vi "mod_AM SSB CE Demodulation (block processing).vi"(0 "input complex waveform":T5={"t0"=0.0, "dt"=1.0, "Y"=[]} {"Y" format="%.3f"; "dt" format="%^.2e"; "t0" format="%.4f"}, 1 "costas loop parameters":T2={"Alpha"=0.001, "Beta"=2e-05} {"Beta" format="%#_6p"; "Alpha" format="%#_6p"}, 5 "modulation index":dbl=1.0 format="%.2f", 7 "pilot extraction filter":T4={"taps"=81, "approx freq. (Hz)"=0.0, "search (+/- % of Fsampl) "=0.25}, 11 "error in (no error)":errorcluster, 12 "suppress carrier ? (F)":bool, 13 "reset? (T)":bool=TRUE) -> (4 "recovered message signal":dbl[](array[numeric]), 6 "measurements":T3, 8 "filter information":T1 {"Pilot rejection filter"."df" format="%.2p"; "Pilot rejection filter"."f0" format="%.2p"; "Pilot rejection filter"."Mag H(w)" format="%.2p"; "Pilot extraction filter"."df" format="%.2p"; "Pilot extraction filter"."f0" format="%.2p"; "Pilot extraction filter"."Mag H(w)" format="%.2p"}, 15 "error out":errorcluster)   [LabVIEW 2020, in "niAMT.lvlib"]
uses:
  <vilib>/addons/Modulation/niAMT.lvlib
  <vilib>/addons/Modulation/Analog/controls/Complex Data Waveform.ctl
  <vilib>/addons/Modulation/Analog/controls/mod_AM pilot extraction filter.ctl
  <vilib>/addons/Modulation/Analog/controls/mod_AM Measurements.ctl
  <vilib>/addons/Modulation/Analog/controls/mod_Costas loop parameters.ctl
  <vilib>/addons/Modulation/Analog/controls/mod_AM pilot filter info.ctl
  <vilib>/Analysis/baseanly.llb/Mean (DBL).vi
  <vilib>/addons/Modulation/Analog/MT Upconvert Baseband (Real).vi
  <vilib>/Analysis/0measdsp.llb/Scaled Time Domain Window (DBL).vi
  <vilib>/Analysis/NI_AALPro.lvlib
  <vilib>/Analysis/NI_AALBase.lvlib
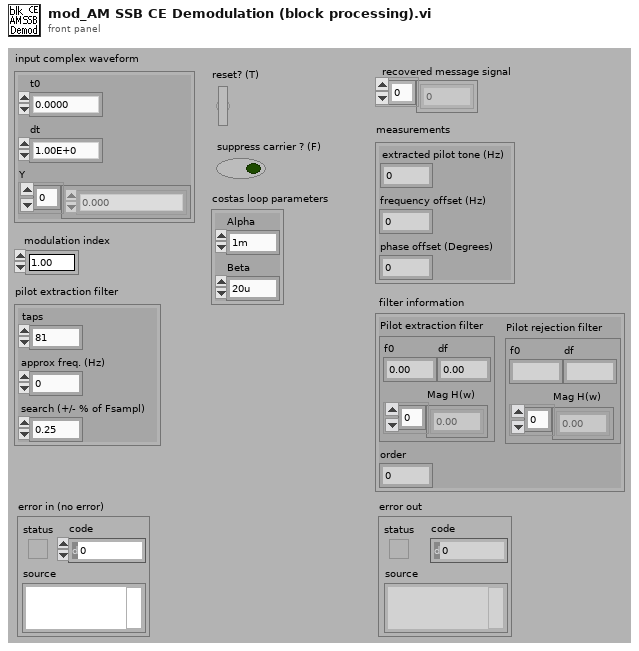
[diagram p1: front panel]
types:
  T1 = typedef "niAMT.lvlib/mod_AM pilot filter info.ctl" = cluster{"Pilot extraction filter":cluster{"f0":dbl, "df":dbl, "Mag H(w)":dbl[]}, "order":i32, "Pilot rejection filter":cluster{"f0":dbl, "df":dbl, "Mag H(w)":dbl[]}}
  T2 = typedef "niAMT.lvlib/mod_Costas loop parameters.ctl" = cluster{"Alpha":dbl, "Beta":dbl}
  T3 = typedef "niAMT.lvlib/mod_AM Measurements.ctl" = cluster{"extracted pilot tone (Hz)":dbl, "phase offset (Degrees)":dbl, "frequency offset (Hz)":dbl}
  T4 = typedef "niAMT.lvlib/mod_AM pilot extraction filter.ctl" = cluster{"taps":i32, "approx freq. (Hz)":dbl, "search (+/- % of Fsampl) ":dbl}
  T5 = typedef "niAMT.lvlib/Complex Data Waveform.ctl" = cluster{"t0":dbl, "dt":dbl, "Y":cdb[]}
  T6 = enum16{"None ", "Hanning", "Hamming", "Blackman-Harris", "Exact Blackman", "Blackman", "Flat Top", "4 Term B-Harris ", "7 Term B-Harris", "Low Sidelobe"}
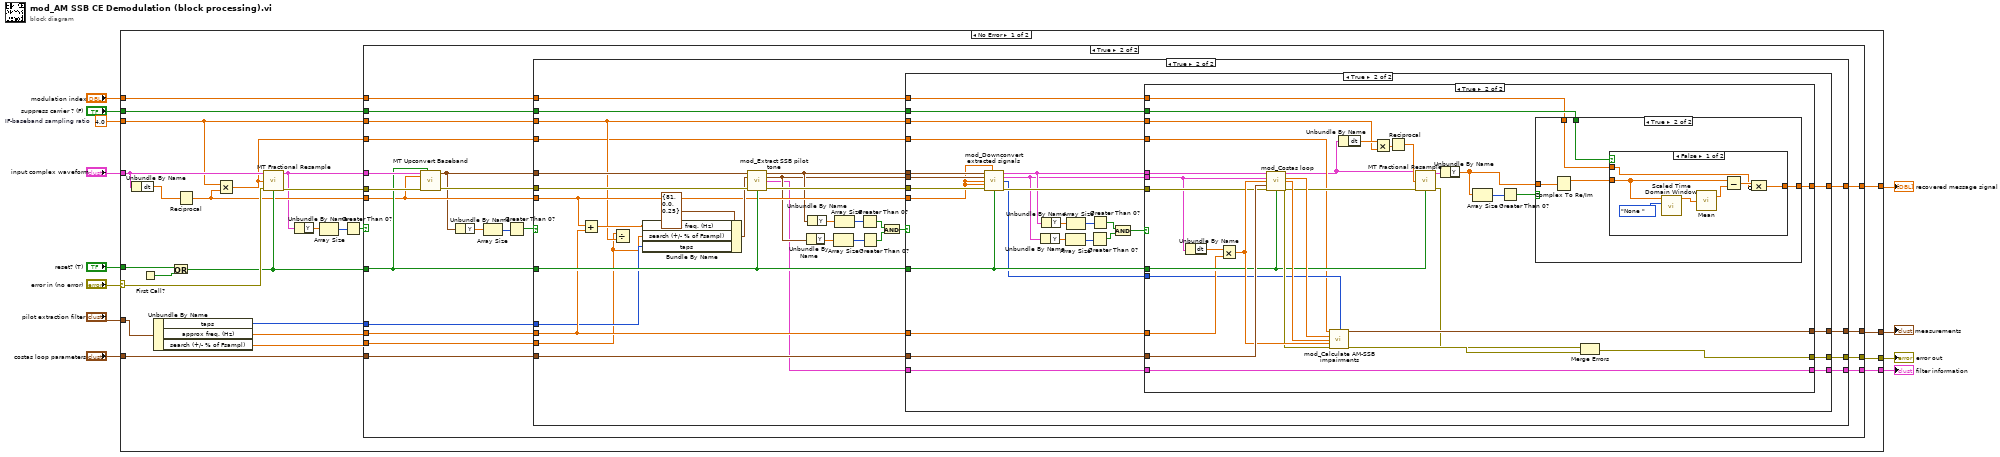
[diagram p0: block diagram]
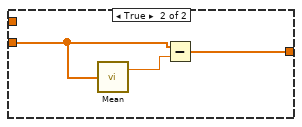
[diagram p7: hidden frame]
diagram:
  w2 = 4.0  # IF-baseband sampling ratio
  n1 = case shown="No Error" "error in (no error)" {
    selector: "error in (no error)" -> [w37 w165]
    tunnel: [w27 w165] -> w11
    tunnel: "input complex waveform" -> [w30 _]
    tunnel: "pilot extraction filter" -> [w32 _]
    tunnel: "reset? (T)" -> [w26 _]
    tunnel: "suppress carrier ? (F)" -> [w35 _]
    tunnel: "modulation index" -> [w34 _]
    tunnel: [w33 _] -> w4
    tunnel: "costas loop parameters" -> [w31 _]
    tunnel: [w29 _] -> w3
    tunnel: w2 -> [w19 _]
    tunnel: [w28 _] -> w1
    frame No Error {
      n2 = Unbundle By Name(w30) -> ("dt"=w21:dbl)
      n3 = First Call?() -> (First Call?: T/F=w24:bool)
      n4 = Unbundle By Name(w32) -> ("taps"=w17:i32, "approx freq. (Hz)"=w23:dbl, "search (+/- % of Fsampl)"=w22:dbl)
      n5 = Or(x=w26, y=w24) -> (x .or. y?=w25:bool)
      n6 = Reciprocal(x=w21) -> (1/x=w20:dbl)
      n7 = Multiply(x=w19, y=w20) -> (x*y=w18:dbl)
      n8 = call <vilib>:"MT Fractional Resample.vi"("input complex waveform"=w30, "desired sample rate (Hz)"=w18, "error in (no error)"=w37, "reset? (T)"=w25) -> ("output complex waveform"=w16:T5, "error out"=w36:errorcluster)  [unwired: 1 in, 9 out]
      n9 = Unbundle By Name(w16) -> ("Y"=w15:cdb[])
      n10 = Array Size(array=w15) -> (size(s)=w14:i32)
      n11 = Greater Than 0?(x=w14) -> (x > 0?=w13:bool)
      n12 = case shown="True" w13 {
        tunnel: w36 -> [w38 w59]
        tunnel: w35 -> [_ w58]
        tunnel: w34 -> [_ w57]
        tunnel: [_ w56] -> w33
        tunnel: w31 -> [_ w54]
        tunnel: w16 -> [_ w53]
        tunnel: [_ w52] -> w29
        tunnel: [_ w51] -> w28
        tunnel: [w38 w50] -> w27
        tunnel: w25 -> [_ w49]
        tunnel: w23 -> [_ w48]
        tunnel: w22 -> [_ w47]
        tunnel: w20 -> [_ w46]
        tunnel: w19 -> [_ w45]
        tunnel: w18 -> [_ w44]
        tunnel: w17 -> [_ w43]
        frame False {
          # "NOTE: Do not perform any processing, since input array sizes are zero-sized"
        }
        frame True {
          n13 = call-poly <vilib>:"MT Upconvert Baseband.vi"("baseband waveform (complex)"=w53, "reset? (F)"=w49, "carrier frequency (Hz)"=w46, "error in (no error)"=w59) -> ("passband waveform"=w41:waveform(dbl), "error out"=w55:errorcluster)  [unwired: 10 out]
          n14 = Unbundle By Name(w41) -> ("Y"=w40:dbl[])
          n15 = Array Size(array=w40) -> (size(s)=w42:i32)
          n16 = Greater Than 0?(x=w42) -> (x > 0?=w39:bool)
          n17 = case shown="True" w39 {
            tunnel: w58 -> [_ w90]
            tunnel: w57 -> [_ w89]
            tunnel: [_ w88] -> w56
            tunnel: w55 -> [w60 w87]
            tunnel: w54 -> [_ w86]
            tunnel: w41 -> [_ w84]
            tunnel: [_ w62] -> w52
            tunnel: [_ w83] -> w51
            tunnel: [w60 w82] -> w50
            tunnel: w49 -> [_ w79]
            tunnel: w48 -> [_ w78]
            tunnel: w47 -> [_ w61]
            tunnel: w46 -> [_ w77]
            tunnel: w45 -> [_ w76]
            tunnel: w44 -> [_ w75]
            tunnel: w43 -> [_ w73]
            frame False {
              # "NOTE: Do not perform any processing, since input array sizes are zero-sized"
            }
            frame True {
              n18 = Add(x=w77, y=w78) -> (x+y=w80:dbl)
              n19 = Divide(x=w61, y=w76) -> ()  [unwired: 1 out]
              n20 = Bundle By Name(cluster=T4 {"taps"=81, "approx freq. (Hz)"=0.0, "search (+/- % of Fsampl) "=0.25} ("pilot extraction filter"), "approx freq. (Hz)"=w80, "search (+/- % of Fsampl)"=w61, "taps"=w73) -> (w85:T4)
              n21 = call <vilib>:"mod_Extract SSB pilot tone.vi"("passband waveform"=w84, "pilot extraction filter"=w85, "error in (no error)"=w87, "reset? (T)"=w79) -> ("extracted AM modulated wfm (IF)"=w71:waveform(dbl), "extracted pilot tone wfm (IF)"=w69:waveform(dbl), "filter information"=w63:T1, "error out"=w81:errorcluster)  [unwired: 8 out]
              n22 = Unbundle By Name(w69) -> ("Y"=w70:dbl[])
              n23 = Unbundle By Name(w71) -> ("Y"=w72:dbl[])
              n24 = Array Size(array=w70) -> (size(s)=w67:i32)
              n25 = Array Size(array=w72) -> (size(s)=w68:i32)
              n26 = Greater Than 0?(x=w68) -> (x > 0?=w66:bool)
              n27 = Greater Than 0?(x=w67) -> (x > 0?=w65:bool)
              n28 = And(x=w66, y=w65) -> (x .and. y?=w64:bool)
              n29 = case shown="True" w64 {
                tunnel: w90 -> [_ w118]
                tunnel: w89 -> [_ w117]
                tunnel: [_ w116] -> w88
                tunnel: w86 -> [_ w115]
                tunnel: [_ w114] -> w83
                tunnel: [w91 w113] -> w82
                tunnel: w81 -> [w91 w112]
                tunnel: w71 -> [_ w111]
                tunnel: w69 -> [_ w110]
                tunnel: w79 -> [_ w109]
                tunnel: w78 -> [_ w107]
                tunnel: w77 -> [_ w105]
                tunnel: w76 -> [_ w104]
                tunnel: w75 -> [_ w103]
                tunnel: w63 -> [_ w101]
                tunnel: [_ w102] -> w62
                frame False {
                  # "NOTE: Do not perform any processing, since input array sizes are zero-sized"
                }
                frame True {
                  n30 = call <vilib>:"mod_Downconvert extracted signals.vi"("extracted AM modulated wfm (IF)"=w111, "carrier frequency"=w105, "extracted pilot tone wfm (IF)"=w110, "passband bandwidth (AM modulated wfm)"=w105, "passband bandwidth (pilot tone wfm)"=w105, "error in (no error)"=w112, "reset? (T)"=w109) -> ("extracted AM modulated signal (baseband)"=w98:cluster{"t0":dbl, "dt":dbl, "Y":cdb[]}, "extracted pilot tone (baseband)"=w95:cluster{"t0":dbl, "dt":dbl, "Y":cdb[]}, "downconversion filter length"=w106:i32, "error out"=w108:errorcluster)  [unwired: 5 out]
                  n31 = Unbundle By Name(w95) -> ("Y"=w96:cdb[])
                  n32 = Unbundle By Name(w98) -> ("Y"=w100:cdb[])
                  n33 = Array Size(array=w96) -> (size(s)=w97:i32)
                  n34 = Array Size(array=w100) -> (size(s)=w99:i32)
                  n35 = Greater Than 0?(x=w97) -> (x > 0?=w93:bool)
                  n36 = Greater Than 0?(x=w99) -> (x > 0?=w94:bool)
                  n37 = And(x=w94, y=w93) -> (x .and. y?=w92:bool)
                  n38 = case shown="True" w92 {
                    tunnel: w118 -> [_ w147]
                    tunnel: w117 -> [_ w146]
                    tunnel: [_ w145] -> w116
                    tunnel: w115 -> [_ w144]
                    tunnel: [_ w137] -> w114
                    tunnel: [w119 w134] -> w113
                    tunnel: w109 -> [_ w132]
                    tunnel: w108 -> [w119 w131]
                    tunnel: w107 -> [_ w130]
                    tunnel: w106 -> [_ w129]
                    tunnel: w104 -> [_ w128]
                    tunnel: w103 -> [_ w127]
                    tunnel: w98 -> [_ w126]
                    tunnel: w95 -> [_ w125]
                    tunnel: [_ w123] -> w102
                    tunnel: w101 -> [_ w123]
                    frame False {
                      # "NOTE: Do not perform any processing, since input array sizes are zero-sized"
                    }
                    frame True {
                      n39 = Unbundle By Name(w125) -> ("dt"=w133:dbl)
                      n40 = Multiply(x=w133, y=w130) -> (x*y=w139:dbl)
                      n41 = call <vilib>:"mod_Costas loop.vi"("extracted AM modulated signal"=w126, "extracted pilot tone"=w125, "pilot tone"=w139, "costas loop parameters"=w144, "error in (no error)"=w131, "reset? (T)"=w132) -> ("recovered AM modulated signal"=w124:cluster{"t0":dbl, "dt":dbl, "Y":cdb[]}, "frequency offset"=w141:dbl, "phase offset (degrees)"=w140:dbl, "error out"=w138:errorcluster)  [unwired: 6 out]
                      n42 = call <vilib>:"mod_Calculate AM-SSB impairments.vi"("IF sampling frequency"=w127, "downconversion filter length"=w129, "frequency offset (normalized)"=w141, "phase offset (degrees)"=w140, "approx. pilot tone (normalized)"=w139, "error in (no error)"=w138) -> ("measurements"=w137:T3, "error out"=w136:errorcluster)  [unwired: 8 out]
                      n43 = Unbundle By Name(w124) -> ("dt"=w142:dbl)
                      n44 = Multiply(x=w142, y=w128) -> (x*y=w149:dbl)
                      n45 = Reciprocal(x=w149) -> (1/x=w148:dbl)
                      n46 = call <vilib>:"MT Fractional Resample.vi"("input complex waveform"=w124, "desired sample rate (Hz)"=w148, "error in (no error)"=w138, "reset? (T)"=w132) -> ("output complex waveform"=w143:T5, "error out"=w135:errorcluster)  [unwired: 1 in, 9 out]
                      n47 = Unbundle By Name(w143) -> ("Y"=w122:cdb[])
                      n48 = Array Size(array=w122) -> (size(s)=w121:i32)
                      n49 = Greater Than 0?(x=w121) -> (x > 0?=w120:bool)
                      n50 = case shown="True" w120 {
                        tunnel: w147 -> [_ w153]
                        tunnel: w146 -> [_ w152]
                        tunnel: [_ w151] -> w145
                        tunnel: w122 -> [_ w150]
                        frame False {
                          # "NOTE: Do not perform any processing, since input array sizes are zero-sized"
                        }
                        frame True {
                          n51 = Complex To Re/Im(x + iy=w150) -> (x=w154:dbl[])  [unwired: 1 out]
                          n52 = case shown="False" w153 {
                            tunnel: [w157 w163] -> w151
                            tunnel: w154 -> [w155 w162]
                            tunnel: w152 -> [w156 _]
                            frame False {
                              n53 = call-poly <vilib>:"Scaled Time Domain Window.vi"("window"=T6."None ", "X"=w155) -> ("Windowed X"=w160:dbl[])  [unwired: 1 in, 8 out]
                              n54 = call-poly <vilib>:"Mean.vi"("X"=w160) -> ("mean"=w158:dbl)  [unwired: 1 out]
                              n55 = Subtract(x=w155, y=w158) -> (x-y=w159:dbl[])
                              n56 = Compound Arithmetic op=MULTIPLY(w159, invert w156) -> (w157:dbl[])
                            }
                            frame True {
                              n57 = call-poly <vilib>:"Mean.vi"("X"=w162) -> ("mean"=w164:dbl)  [unwired: 1 out]
                              n58 = Subtract(x=w162, y=w164) -> (x-y=w163:dbl[])
                            }
                          }
                        }
                      }
                      n59 = Merge Errors(w135, w136) -> (w134:errorcluster)
                    }
                  }
                }
              }
            }
          }
        }
      }
    }
    frame Error {
    }
  }
  "error out" <- w11
  "recovered message signal" <- w4
  "measurements" <- w1
  "filter information" <- w3
